vi "helloworld.vi"() -> (2 "Output":string)   [LabVIEW 2014]
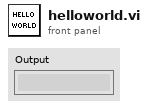
[diagram p1: front panel]
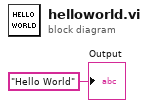
[diagram p0: block diagram]
diagram:
  "Output" <- "Hello World" ("Output")
